vi "Continuous MeasSubVi.vi"(0 "GPIB in":string="18", 4 "setup":T1 {"delay (s)" min=0 max=25.5 step=0.1 format="%.1f"; "sample interval (s)" min=1.1 max=99999.9 step=0.1 format="%.1f"; "longest wavelength" min=190 max=820 step=1; "shortest wavelength" min=190 max=820 step=1; "integration time (s)" min=0.1 max=25.5 step=0.1 format="%.1f"}) -> (5 "processor time used":sgl format="%.2f", 6 "GPIB out":string="18", 7 "measurement":dbl[](array[numeric])=[-4.07142, -4.08921, -4.05722, -4.06889, -4.04566, -4.12405, -4.10371, -4.10472, -4.01449, -4.05473, -4.09877, -3.95974, -3.98947, -3.99844, -3.98602, -3.95837, -4.10552, -4.07749, -4.0634, -4.06492, -4.08459, -4.11593, -3.97463, -4.01223, -4.04632, -4.07437, -4.09077, -4.09436, -4.08288, -4.05764, -4.02265, -3.97798, -4.11219, -4.07209, -4.03381, -4.11972, -4.10028, -4.09083, -4.09074, -4.09916, -4.11592, -4.02854, -4.05818, -4.09405, -4.12223, -3.9674, -3.98504, -3.98738, -3.984, -3.99179, -3.97789, -3.97294, -3.9582, -4.11819, -4.10696, -4.09436, -4.08184, -4.06178, -4.06657, -4.06227, -4.06236, -4.06544, -4.06669, -4.07881, -4.08798, -4.10186, -4.1157, -3.95091, -3.96565, -3.97851, -3.99177, -4.00169, -4.01187, -4.01802, -4.02114, -4.022, -4.01861, -4.01106, -4.00169, -3.98953, -3.96856, -3.94934, -4.10746, -4.08482, -4.06143, -4.0386, -4.01271, -4.12512, -4.06634, -4.11845, -4.10632, -4.10354, -4.11137, -4.12138, -4.05122, -4.05436, -4.05596, -4.05645, -4.06637, -4.08909, -4.07978, -4.12355, -4.11839, -4.12402, -4.05502, -4.0211, -4.01951, -4.04148, -4.03601, -4.03636, -4.0373, -4.05973, -4.06129, -4.05668, -4.05848, -4.09931, -3.95468, -4.10307, -4.07867, -4.09898, -3.96177, -4.06494, -4.08384, -4.0715, -4.0635, -4.07588, -4.10095, -4.08938, -4.07307, -4.04325, -4.01689, -4.10592, -4.08406, -4.07919, -4.10508, -4.07077, -4.11323, -4.08508, -4.1238, -4.06275, -4.07011, -4.09667, -4.1103, -4.09436, -4.09423, -4.11277, -4.11914, -4.10025, -4.11897, -4.07615, -4.0525, -4.10298, -4.08853, -4.10641, -4.09167, -4.0884, -4.1054, -4.1212, -4.10984, -4.1269, -4.1181, -4.09352, -4.10942, -4.10719, -4.09541, -4.10539, -4.09744, -4.10363, -4.10733, -4.08645, -4.11087, -4.10862, -4.10768, -4.10115, -4.11785, -4.10997, -4.0973, -4.10836, -4.09333, -4.12327, -4.10113, -4.12153, -4.10049, -4.10392, -4.10408, -4.1145, -4.09075, -4.06936, -4.06338, -4.04913, -4.03273, -4.05108, -3.8739, -3.90065, -3.88583, -3.95143, -3.87205, -3.88571, -4.12011, -4.07241, -3.96221, -4.12666, -4.08091, -3.97792, -4.07438, -4.07202, -4.06758, -3.97036, -4.12345, -4.0794, -4.09292, -4.06901, -4.08995, -4.11099, -4.05725, -4.09049, -4.06442, -4.09991, -4.08151, -4.11541, -4.11535, -4.11039, -4.11004, -4.11598, -4.09898, -4.12492, -4.06416, -4.05345, -4.02876, -4.09939, -4.10003, -4.11239, -4.08584, -3.95483, -4.08033, -4.08735, -4.10513, -4.0442, -3.94911, -3.94268, -4.00511, -4.09843, -3.97695, -3.99497, -4.10845, -4.10839, -4.05577, -4.09848, -4.10217, -4.1099, -4.10643, -4.11563, -4.08067, -4.11073, -4.09977, -4.01991, -4.07026, -3.99772, -4.09307, -4.11843, -4.10134, -4.08406, -4.11689, -4.04159, -4.0987, -4.09939, -4.06648, -4.10064, -4.10548, -4.12437, -4.10772, -4.12313, -4.09571, -4.11756, -4.09054, -4.1108, -4.10881, -4.10511, -4.1157, -4.12921, -4.10816, -4.10789, -4.12104, -4.0986, -4.11882, -4.1145, -4.08699, -4.1203, -4.08033, -4.09431, -4.09814, -4.12849, -4.10231, -4.07093, -4.08964, -4.12213, -4.07734, -4.12287, -4.11428, -4.10539, -4.10459, -4.09613, -4.093, -4.12292, -4.07064, -4.06091, -4.01824, -4.02458, -4.11665, -4.09893, -4.04747, -3.96943, -4.03416, -3.9858, -3.94538, -3.97187] format="%.3e", 8 "error occurred":bool)   [LabVIEW 2015]
uses:
  Continuous settings.ctl
panel:
  out "Absorbance":cluster{"shortest wavelength":sgl, i32, dbl[]}(graph)
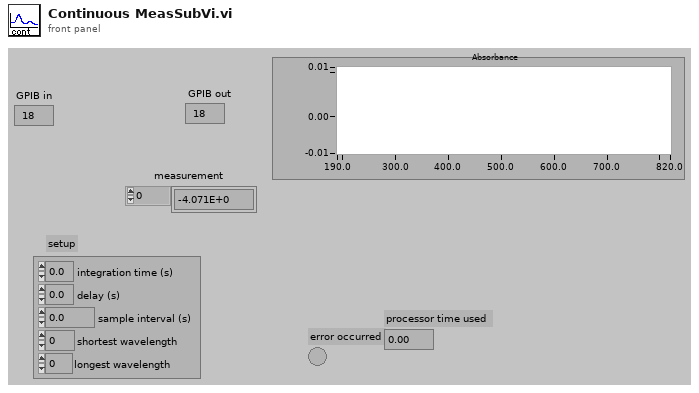
[diagram p1: front panel]
types:
  T1 = typedef "Continuous settings.ctl" = cluster{"integration time (s)":sgl, "shortest wavelength":sgl, "longest wavelength":sgl, "sample interval (s)":dbl, "delay (s)":sgl}
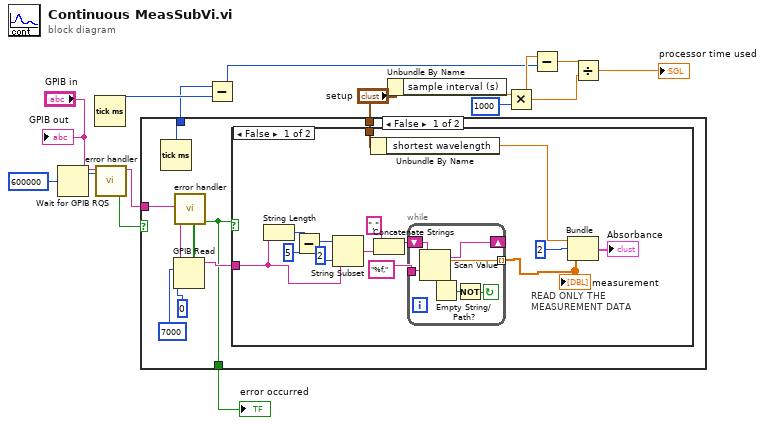
[diagram p0: block diagram]
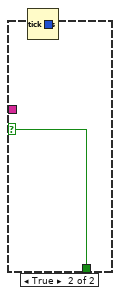
[diagram p3: hidden frame]
diagram:
  n1 = Wait for GPIB RQS(3:600000 ("timeout ms (488.2 global)"), 4:"GPIB in") -> (1:w13:i16)  [unwired: 1 in, 1 out]
  n2 = Tick Count (ms)() -> (millisecond timer value=w10:u32)
  n3 = call "error handler.vi"("poll response"=w13, "GPIB in"="GPIB in") -> ("error occurred"=w12:bool, "GPIB out"=w14:string)  [unwired: 3 in, 1 out]
  n4 = case shown="False" w12 {
    selector: w12 -> [_ w45]
    tunnel: w14 -> [w19 _]
    tunnel: [w18 w45] -> w11
    tunnel: [w17 w44] -> w9
    tunnel: "setup" -> [w16 _]
    frame False {
      n5 = Tick Count (ms)() -> (millisecond timer value=w17:u32)
      n6 = GPIB Read(0:w19, 1:7000, 2:0) -> (5:w21:string, 6:w20:bool[])  [unwired: 2 in, 1 out]
      n7 = call "error handler.vi"("status array"=w20, "GPIB in"=w19) -> ("error occurred"=w18:bool)  [unwired: 3 in, 2 out]
      n8 = case shown="False" w18 {
        tunnel: w21 -> [w27 _]
        tunnel: w16 -> [w26 _]
        frame False {
          # "READ ONLY THE MEASUREMENT DATA"
          n9 = String Length(string=w27) -> (length=w32:i32)
          n10 = Subtract(x=w32, y=5) -> (x-y=w33:i32)
          n11 = String Subset(string=w27, offset (0)=2, length (rest)=w33) -> (substring=w34:string)
          n12 = Unbundle By Name(w26) -> ("shortest wavelength"=w25:sgl)
          n13 = Concatenate Strings(w34, ",") -> (w29:string)
          n14 = while {
            tunnel: "%f," -> [w38]
            tunnel: [w42] -> w36 mode=indexing
            shift-left: w29 -> [w41]
            shift-right: [w40] -> _
            stop <- w43 continue-if-true
            n15 = Scan Value(string=w41, format string=w38) -> (output string=w40:string, value=w42:dbl)  [unwired: 1 in]
            n16 = Empty String/Path?(string/path=w40) -> (empty?=w39:bool)
            n17 = Not(x=w39) -> (.not. x?=w43:bool)
          }
          "measurement" <- w36
          n18 = Bundle("shortest wavelength"=w25, 2, w36) -> (→"Absorbance":cluster{"shortest wavelength":sgl, i32, dbl[]})  [unwired: 1 in]
        }
        frame True {
        }
      }
    }
    frame True {
      n19 = Tick Count (ms)() -> (millisecond timer value=w44:u32)
    }
  }
  "error occurred" <- w11
  n20 = Subtract(x=w9, y=w10) -> (x-y=w3:u32)
  n21 = Unbundle By Name("setup") -> ("sample interval (s)"=w7:dbl)
  n22 = Multiply(x=w7, y=1000) -> (x*y=w4:dbl)
  n23 = Subtract(x=w4, y=w3) -> (x-y=w2:dbl)
  n24 = Divide(x=w2, y=w4) -> (x/y=→"processor time used":dbl)
  "GPIB out" <- "GPIB in"
